vi "Creators Creator Queue Alias.vi"(11 "Hello World Event in":refnum<class "Hello World Event.lvclass">) -> (2 "Creator Queue Alias":string, 3 "Hello World Event out":refnum<class "Hello World Event.lvclass">)   [LabVIEW 2021, in "Hello World Event.lvlib" / "Hello World Event.lvclass"]
uses:
  Hello World Event.lvclass
  Hello World Event.lvclass/Hello World Event.ctl
  jettl/Event/Event.lvclass
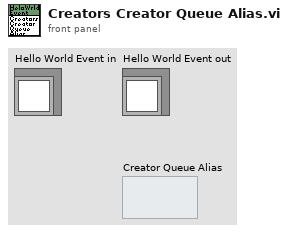
[diagram p1: front panel]
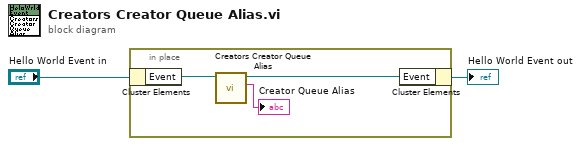
[diagram p0: block diagram]
diagram:
  n1 = in-place {
    n2 = in-place-cluster #1("Hello World Event in") -> ("Event"=w5:refnum<class "Event.lvclass">)
    n3 = call-dynamic "Creators Creator Queue Alias.vi"("Event in"=w5) -> ("Creator Queue Alias"=→"Creator Queue Alias":string, "Event out"=w4:refnum<class "Event.lvclass">)  [unwired: 9 in]
    n4 = in-place-cluster #1("Event"=w4) -> (→"Hello World Event out":refnum<class "Hello World Event.lvclass">)
  }
